vi "initListenFGV.vi"(8 "error in (no error)":errorcluster) -> (0 "error out":errorcluster)   [LabVIEW 2017]
uses:
  TypeDefs/UDPListenFGVCtrl.ctl
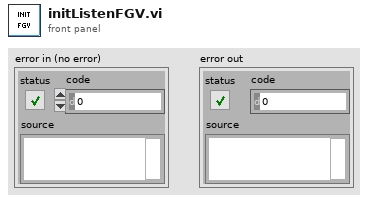
[diagram p1: front panel]
types:
  T1 = typedef "UDPListenFGVCtrl.ctl" = enum16{"Read", "Write"}
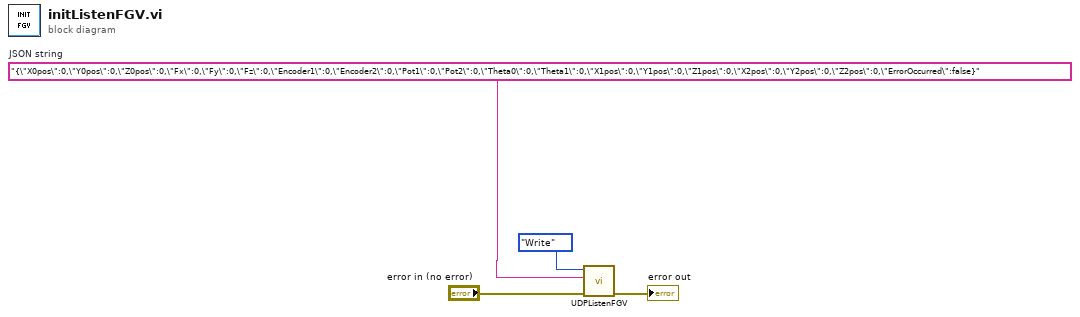
[diagram p0: block diagram]
diagram:
  w1 = "{\"X0pos\":0,\"Y0pos\":0,\"Z0pos\":0,\"Fx\":0,\"Fy\":0,\"Fz\":0,\"Encoder1\":0,\"Encoder2\":0,\"Pot1\":0,\"Pot2\":0,\"Theta0\":0,\"Theta1\":0,\"X1pos\":0,\"Y1pos\":0,\"Z1pos\":0,\"X2pos\":0,\"Y2pos\":0,\"Z2pos\":0,\"ErrorOccurred\":false}"  # JSON string
  n1 = call "UDPListenFGV.vi"("error in (no error)"="error in (no error)", "Write Data"=w1, "Enum"=UDPListenFGVCtrl."Write") -> ("error out"=→"error out":errorcluster)  [unwired: 7 in, 1 out]
